vi "盐度补偿值写入.vi"(8 "Error in":errorcluster caption="Error in (no error)", 10 "盐度补偿值":sgl, 11 "MB session in":refnum<class "MB_Master.lvclass">) -> (0 "error out":errorcluster, 3 "MB session out":refnum<class "MB_Master.lvclass">)   [LabVIEW 2016, in "斯坦道氨氮.lvlib"]
uses:
  <vilib>/Plasmionique/MB Master/MB_Master/MB_Master.lvclass
  <vilib>/Plasmionique/MB Master/MB Master.lvlib
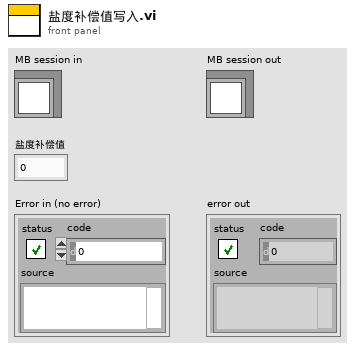
[diagram p1: front panel]
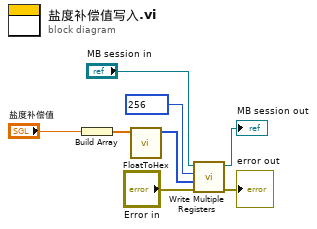
[diagram p0: block diagram]
diagram:
  n1 = Build Array("盐度补偿值") -> (w2:sgl[])
  n2 = call "FloatToHex.vi"("浮点数"=w2) -> ("DCBA整形输出"=w1:u16[])  [unwired: 10 in]
  n3 = call <vilib>:"Write Multiple Registers.vi"("error in (no error)"="Error in", "values"=w1, "starting address"=u16 256, "MB session in"="MB session in") -> ("error out"=→"error out":errorcluster, "MB session out"=→"MB session out":refnum<class "MB_Master.lvclass">)  [unwired: 6 in]
